vi "Initialize.vi"(7 "not in use":string="Setpoint.ch%d.SP", 8 "error in":errorcluster, 9 "Number of Channels":u32=1, 10 "Instance Name":string, 11 "Current Actual Value in":refnum<class "Current Actual Value.lvclass">) -> (0 "error out":errorcluster, 3 "Current Actual Value out":refnum<class "Current Actual Value.lvclass">)   [LabVIEW 2023, in "Current Actual Value.lvclass"]
uses:
  Current Actual Value.lvclass
  Current Actual Value.lvclass/Current Actual Value.ctl
  Actual Value/Actual Value.lvclass
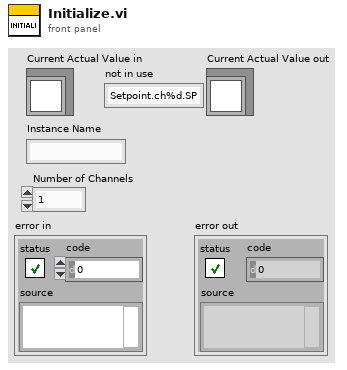
[diagram p1: front panel]
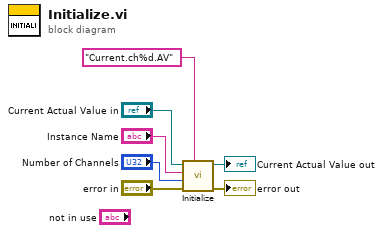
[diagram p0: block diagram]
diagram:
  n1 = call-parent "Initialize.vi"("ChannelName"="Current.ch%d.AV", "error in"="error in", "Number of Channels"="Number of Channels", "Instance Name"="Instance Name", "Actual Value in"="Current Actual Value in") -> ("error out"=→"error out":errorcluster, "Actual Value out"=→"Current Actual Value out":refnum<class "Current Actual Value.lvclass">)  [unwired: 5 in]
